vi "AUTON_Write_Version.vi"(10 "Current File":dbl, 11 "Auton Files":string[](array[string])) -> ()   [LabVIEW 2012]
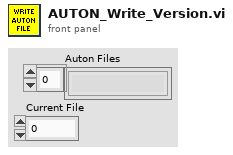
[diagram p1: front panel]
types:
  T1 = enum16{"open", "replace", "create", "open or create", "replace or create", "replace or create with confirmation"}
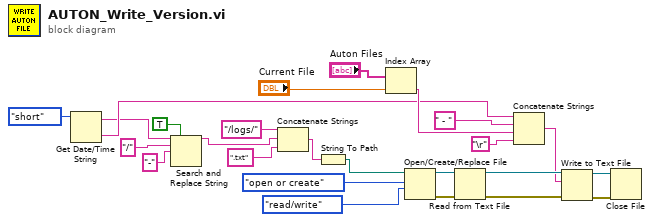
[diagram p0: block diagram]
diagram:
  n1 = Get Date/Time String(date format (0)=enum16{"short", "long", "abbreviated"}."short") -> (date string=w16:string, time string=w22:string)  [unwired: 2 in]
  n2 = Search and Replace String(replace all?=TRUE ("replace all? (F)"), input string=w16, search string="/", replace string="-" ("replace string (\"\")")) -> (result string=w20:string)  [unwired: 4 in, 3 out]
  n3 = Concatenate Strings("/logs/" ("string"), w20, ".txt" ("string")) -> (w14:string)
  n4 = String To Path(string=w14) -> (path=w12:path)
  n5 = Index Array(array="Auton Files", index="Current File") -> (element=w25:string)
  n6 = Open/Create/Replace File(file path (use dialog)=w12, operation (0:open)=T1."open or create", access (0:read/write)=enum16{"read/write", "read-only", "write-only"}."read/write") -> (refnum out=w6:refnum<file>, error out=w5:errorcluster)  [unwired: 3 in, 1 out]
  n7 = Read from Text File(file (use dialog)=w6, error in=w5) -> (refnum out=w3:refnum<file>, error out=w2:errorcluster)  [unwired: 2 in, 2 out]
  n8 = Concatenate Strings(w22, " - " ("string"), w25, "\r") -> (w1:string)
  n9 = Write to Text File(file (use dialog)=w3, text=w1, error in=w2) -> (refnum out=w11:refnum<file>, error out=w10:errorcluster)  [unwired: 1 in, 1 out]
  n10 = Close File(refnum=w11, error in=w10) -> ()  [unwired: 2 out]
